vi "Allgemein_Data_By_Keys.vi"(10 "String":string[][](array[string]), 11 "Keys (Eingang)":string[](array[string])) -> (2 "Length Array  (Ausgang)":i32[](array[numeric]), 3 "Array (Ausgang)":string[][][](array[string]))   [LabVIEW 2020, in "System Einstellungen V2.lvlib"]
doc: "Gibt die Einträge zu den Schlüssel (Keys wie [Optionen], [Gasteiler ...] aus einer Textdatei separat wieder.\nDie Einzelnen Arrays müssen danach noch mit dem Length Array auf die tatsächliche Länge zurück gestutzt werden, da im mehrdimensionalen alle die selbe Länge haben !\nEs dürfen aber (drezeit noch) keine Keys ausgelassen werden, dahinter können noch welche sein !\nDie Reihenfolge der Schlüsselpositionen in der Datei ist egal.\nEingang: String aus Datei als 2D Array (erste Spalte enthält die keys), Keys die ausgelesen werden sollen als Array.\nAusgang: 3D Array mit den Einträgen, Length Array zum zurück stutzen auf die tatsächliche Länge\nRIW, 2022-12-13"
uses:
  System Einstellungen V2.lvlib
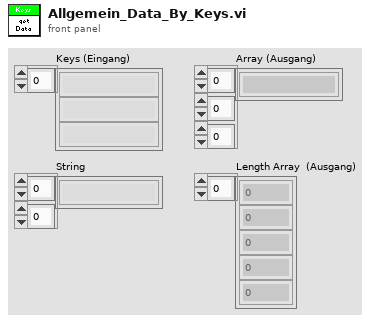
[diagram p1: front panel]
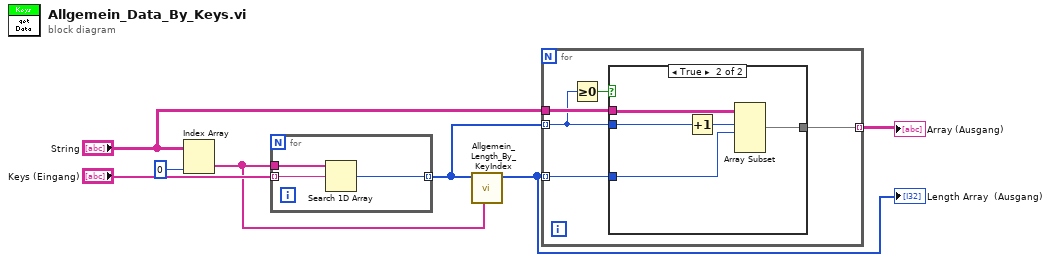
[diagram p0: block diagram]
diagram:
  n1 = Index Array(array="String", index (col)=0 ("Deaktivierter Index (Spalte)")) -> (element=w1:string[])  [unwired: 1 in]
  n2 = for {
    tunnel: w1 -> [w10]
    tunnel: "Keys (Eingang)" -> [w9] mode=indexing
    tunnel: [w8] -> w4 mode=indexing
    n3 = Search 1D Array(1D array=w10, element=w9) -> (index of element=w8:i32)  [unwired: 1 in]
  }
  n4 = call "Allgemein_Length_By_KeyIndex.vi"("Teil-Array"=w1, "Key Index Array (Eingang)"=w4) -> ("Length Array  (Ausgang)"=w5:i32[])  [unwired: 6 in, 3 out]
  "Length Array  (Ausgang)" <- w5
  n5 = for {
    tunnel: "String" -> [w14]
    tunnel: [w13] -> w2 mode=indexing
    tunnel: w5 -> [w12] mode=indexing
    tunnel: w4 -> [w11] mode=indexing
    n6 = Greater Or Equal To 0?(x=w11) -> (x >= 0?=w15:bool)
    n7 = case shown="True" w15 {
      tunnel: [_ w20] -> w13
      tunnel: w12 -> [_ w19]
      tunnel: w14 -> [_ w18]
      tunnel: w11 -> [_ w17]
      frame False {
      }
      frame True {
        n8 = Increment(x=w17) -> (x+1=w16:i32)
        n9 = Array Subset(array=w18, index (row)=w16, length (row)=w19) -> (w20:string[][])  [unwired: 2 in]
      }
    }
  }
  "Array (Ausgang)" <- w2
